vi "Make Switch.vi"(7 "State (0: ssNone)":i32(ring) items=["ssNone", "ssA", "ssB"], 8 "error in (no error)":errorcluster, 9 "Physical Channel (1)":i32=1, 10 "Name (\"\")":string="\"\"", 11 "VISA resource name":refnum<visa-resource-name>) -> (0 "error out":errorcluster, 3 "VISA resource name out":refnum<visa-resource-name>)   [LabVIEW 2014, in "Stanford Research SR1.lvlib"]
doc: "Connects the physical channel (1-12) of the named switch to either A,B, or nothing (disconnected)."
uses:
  Stanford Research SR1.lvlib
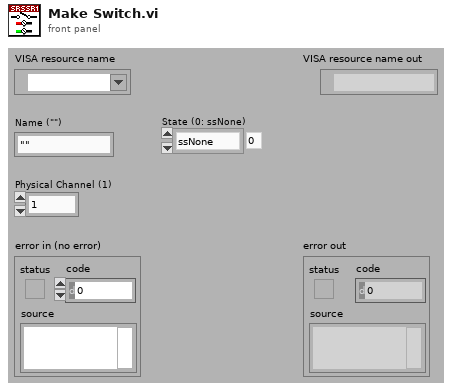
[diagram p1: front panel]
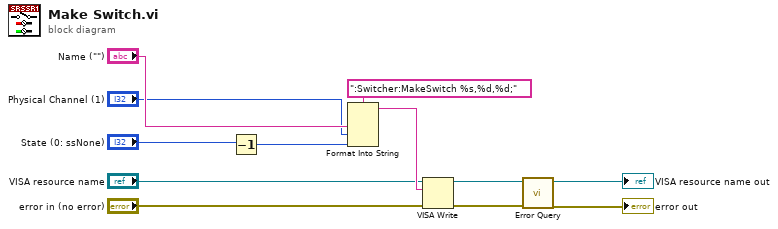
[diagram p0: block diagram]
diagram:
  n1 = Decrement(x="State (0: ssNone)") -> (x-1=w1:i32)
  n2 = Format Into String(format string=":Switcher:MakeSwitch %s,%d,%d;", "Name (\"\")", "Physical Channel (1)", w1) -> (resulting string=w9:string)  [unwired: 2 in, 1 out]
  n3 = VISA Write(VISA resource name="VISA resource name", write buffer=w9, error in (no error)="error in (no error)") -> (VISA resource name out=w6:refnum<visa-resource-name>, error out=w5:errorcluster)  [unwired: 1 out]
  n4 = call "Error Query.vi"("error in (no error)"=w5, "VISA resource name"=w6) -> ("error out"=→"error out":errorcluster, "VISA resource name out"=→"VISA resource name out":refnum<visa-resource-name>)  [unwired: 6 in, 2 out]
